vi "Locate Focal Spot.vi"(11 "Focal Spot":dbl[][](array[numeric])) -> (0 "sy":dbl, 1 "sx":dbl, 2 "cmy":dbl, 3 "cmx":dbl)   [LabVIEW 2014]
uses:
  <vilib>/Analysis/1siggen.llb/Ramp Pattern by Samples.vi
  <vilib>/gmath/interp.llb/Create Mesh Grid (2D) (x,y arrays).vi
  <vilib>/Analysis/NI_AALBase.lvlib
  <vilib>/gmath/NI_Gmath.lvlib
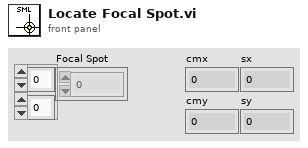
[diagram p1: front panel]
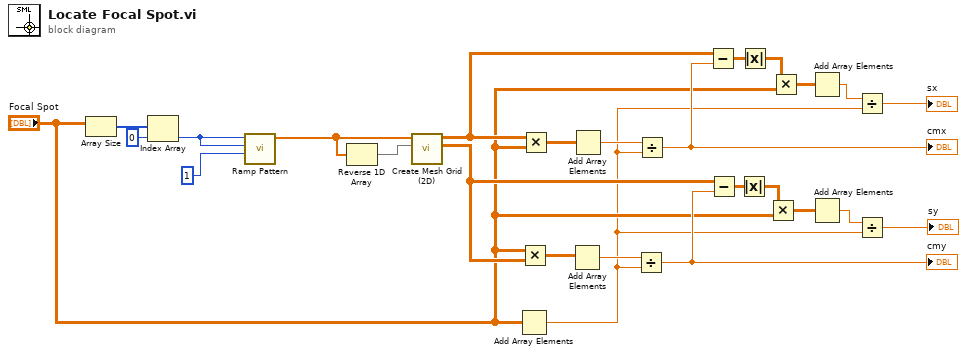
[diagram p0: block diagram]
diagram:
  n1 = Array Size(array="Focal Spot") -> (size(s)=w26:i32[])
  n2 = Index Array(array=w26, index=0) -> (element=w23:i32)
  n3 = call-poly <vilib>:"Ramp Pattern.vi"("start"=1, "end"=w23, "samples"=w23) -> ("Ramp Pattern"=w22:dbl[])  [unwired: 7 in, 1 out]
  n4 = Reverse 1D Array(array=w22) -> (reversed array=w21:dbl[])
  n5 = call-poly <vilib>:"Create Mesh Grid (2D).vi"("y domain"=w21, "x domain"=w22) -> ("Y"=w11:dbl[][], "X"=w16:dbl[][])  [unwired: 7 in, 1 out]
  n6 = Add Array Elements(numeric array="Focal Spot") -> (sum=w6:dbl)
  n7 = Multiply(x="Focal Spot", y=w11) -> (x*y=w19:dbl[][])
  n8 = Multiply(x=w16, y="Focal Spot") -> (x*y=w20:dbl[][])
  n9 = Add Array Elements(numeric array=w19) -> (sum=w17:dbl)
  n10 = Add Array Elements(numeric array=w20) -> (sum=w18:dbl)
  n11 = Divide(x=w17, y=w6) -> (x/y=w10:dbl)
  "cmy" <- w10
  n12 = Divide(x=w18, y=w6) -> (x/y=w15:dbl)
  "cmx" <- w15
  n13 = Subtract(x=w16, y=w15) -> (x-y=w4:dbl[][])
  n14 = Subtract(x=w11, y=w10) -> (x-y=w2:dbl[][])
  n15 = Absolute Value(x=w2) -> (abs(x)=w1:dbl[][])
  n16 = Absolute Value(x=w4) -> (abs(x)=w3:dbl[][])
  n17 = Multiply(x=w1, y="Focal Spot") -> (x*y=w8:dbl[][])
  n18 = Multiply(x=w3, y="Focal Spot") -> (x*y=w14:dbl[][])
  n19 = Add Array Elements(numeric array=w14) -> (sum=w13:dbl)
  n20 = Add Array Elements(numeric array=w8) -> (sum=w7:dbl)
  n21 = Divide(x=w13, y=w6) -> (x/y=→"sx":dbl)
  n22 = Divide(x=w7, y=w6) -> (x/y=→"sy":dbl)
